vi "FunctionErrorCodes.vi"() -> (4 "[user-defined codes]":i32[](array[numeric])=[0, -1, -2, -3, -4, -9, -10], 8 "[user-defined descriptions]":string[](array[string])=["no error", "function error", "communication error", "syntax error", "axis in wrong state", "OWISid chip is not found", "OWISid parameter is empty (not defined)"])   [LabVIEW 2020]
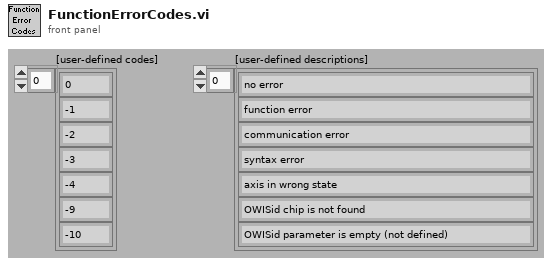
[diagram p1: front panel]
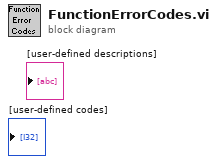
[diagram p0: block diagram]
diagram:
